vi "Pictures.vi"(11 "Pictures":T1) -> (3 "Path":path)   [LabVIEW 2012]
uses:
  pictures.ctl
  <userlib>/_OpenG.lib/file/file.llb/Strip Path - Traditional__ogtk.vi
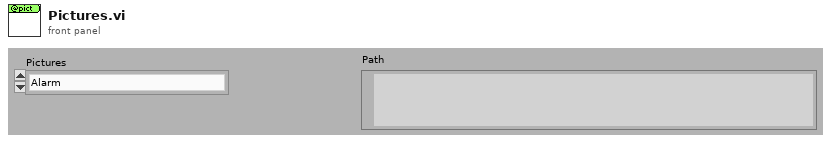
[diagram p1: front panel]
types:
  T1 = typedef "pictures.ctl" = enum16{"Alarm", "Download", "Edition", "Encrypted", "Error", "Hardware Information", "Important", "Memory", "Network", "Package", "Password", "Readme", "Search", "System", "USB", "User", "Wireless", "www"}
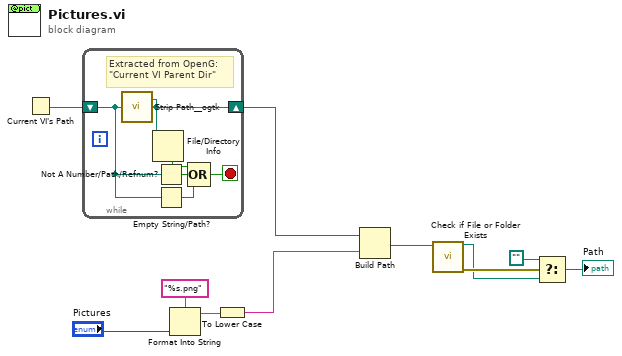
[diagram p0: block diagram]
diagram:
  n1 = Current VI's Path() -> (path=w2:path)
  n2 = while {
    shift-right: [w12] -> w1
    shift-left: w2 -> [w14]
    stop <- w16 stop-if-true
    # "Extracted from OpenG: \n\"Current VI Parent Dir\""
    n3 = call-poly <userlib>:"Strip Path__ogtk.vi"("path"=w14) -> ("stripped path"=w12:path)  [unwired: 1 out]
    n4 = File/Directory Info(path=w12) -> (directory=w17:bool)  [unwired: 1 in, 6 out]
    n5 = Not A Number/Path/Refnum?(number/path/refnum=w14) -> (NaN/Path/Refnum?=w15:bool)
    n6 = Empty String/Path?(string/path=w14) -> (empty?=w13:bool)
    n7 = Compound Arithmetic op=OR(w17, w15, w13) -> (w16:bool)
  }
  n8 = Format Into String(format string="%s.png", "Pictures") -> (resulting string=w9:string)  [unwired: 2 in, 1 out]
  n9 = To Lower Case(string=w9) -> (all lower case string=w8:string)
  n10 = Build Path(base path=w1, name or relative path=w8) -> (appended path=w7:path)
  n11 = call <vilib>:"Check if File or Folder Exists.vi"("path"=w7) -> ("error out"=w6:errorcluster, "dup path"=w5:path)  [unwired: 1 in, 8 out]
  n12 = Select(t=path "", s=w6, f=w5) -> (s? t:f=→"Path":path)
